vi "HW Cleanup.vi"() -> (0 "error out":errorcluster)   [LabVIEW 2013]
uses:
  <vilib>/FPGAPlugInAG/Dynamic/niLvFpga_Close_Dynamic.vi
  <vilib>/rvi/interface/nirviCloseFPGA/nirviCloseFPGA.xnode
  RIG-SPECIFIC FILES/FPGA Refs/FPGA Ref.ctl
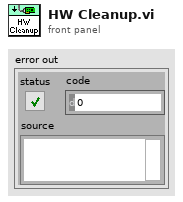
[diagram p1: front panel]
types:
  T1 = typedef "FPGA Ref.ctl" = refnum<k20>
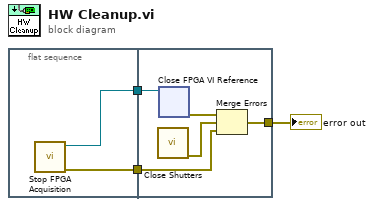
[diagram p0: block diagram]
diagram:
  n1 = flat-sequence {
    tunnel: [w4] -> w2
    tunnel: [w5] -> w1
    tunnel: [w10] -> w3
    tunnel: w2 -> [w7]
    tunnel: w1 -> [w6]
    frame #0 {
      n2 = call "Stop FPGA Acquisition.vi"() -> ("Error Out"=w5:errorcluster, "FPGA Ref"=w4:T1)  [unwired: 10 in]
    }
    frame #1 {
      n3 = call "Close Shutters.vi"() -> ("error out (no error)"=w8:errorcluster)  [unwired: 11 in]
      n4 = xnode ("Close FPGA VI Reference")("FPGA VI Reference In"=w7) -> ("error out"=w9:errorcluster)  [unwired: 1 in]
      n5 = Merge Errors(w9, w8, w6) -> (w10:errorcluster)
    }
  }
  "error out" <- w3
